vi "TestLoop ReadDataAndSwitchBuffers.vi"() -> ()   [LabVIEW 2013]
uses:
  My circular buffer info.ctl
panel:
  out "buffer size (in bytes)":i64
  out "Buffer offset (in bytes)":i64
  out "element read buffer Q":refnum<file>
  out "elements of read buffer Q":refnum<file>[](array[refnum])
  out "# elements in read buffer Q":i32
  out "element command Q":enum16{"toggle buffers", "data event", "stop"}(ring)
  out "elements command Q":enum16{"toggle buffers", "data event", "stop"}[](array[ring])
  out "# elements in command Q":i32
  in  "stop":bool
  in  "buffer2 path":path
  in  "buffer1 path":path
  in  "archive directory":path
  in  "num blocks  prior":i32
  in  "num blocks after":i32
  in  "bytes/sample":i32
  in  "samples/block/channel":i32
  in  "number of channels":i32
  out "write pointer (block position)":i32
  out "Waveform Graph":i16[][](graph)
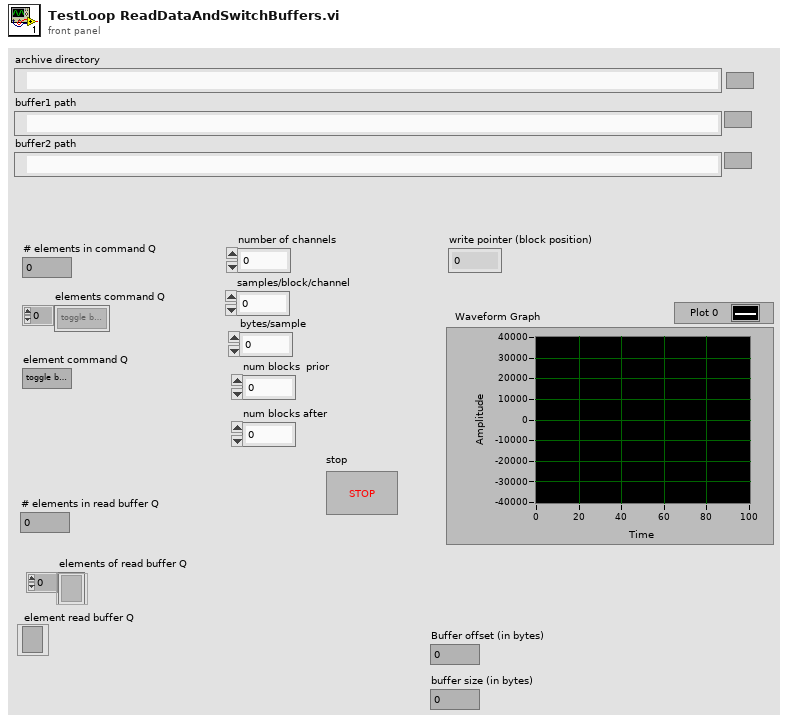
[diagram p1: front panel]
types:
  T1 = typedef "My circular buffer info.ctl" = cluster{"buff ref1":refnum<file>, "buff ref2":refnum<file>, "buffer1 path":path, "buffer2 path":path, "archive directory":path, "xml header":string, "num blocks  prior":i32, "num blocks after":i32, "blocks/event":i32, "samples/block":i32, "bytes/sample":i32, "number of channels":i32, "samples/block/channel":i32, "read buffer ref queue":refnum<queue>, "Event delay queue":refnum<queue>, "command queue":refnum<queue>}
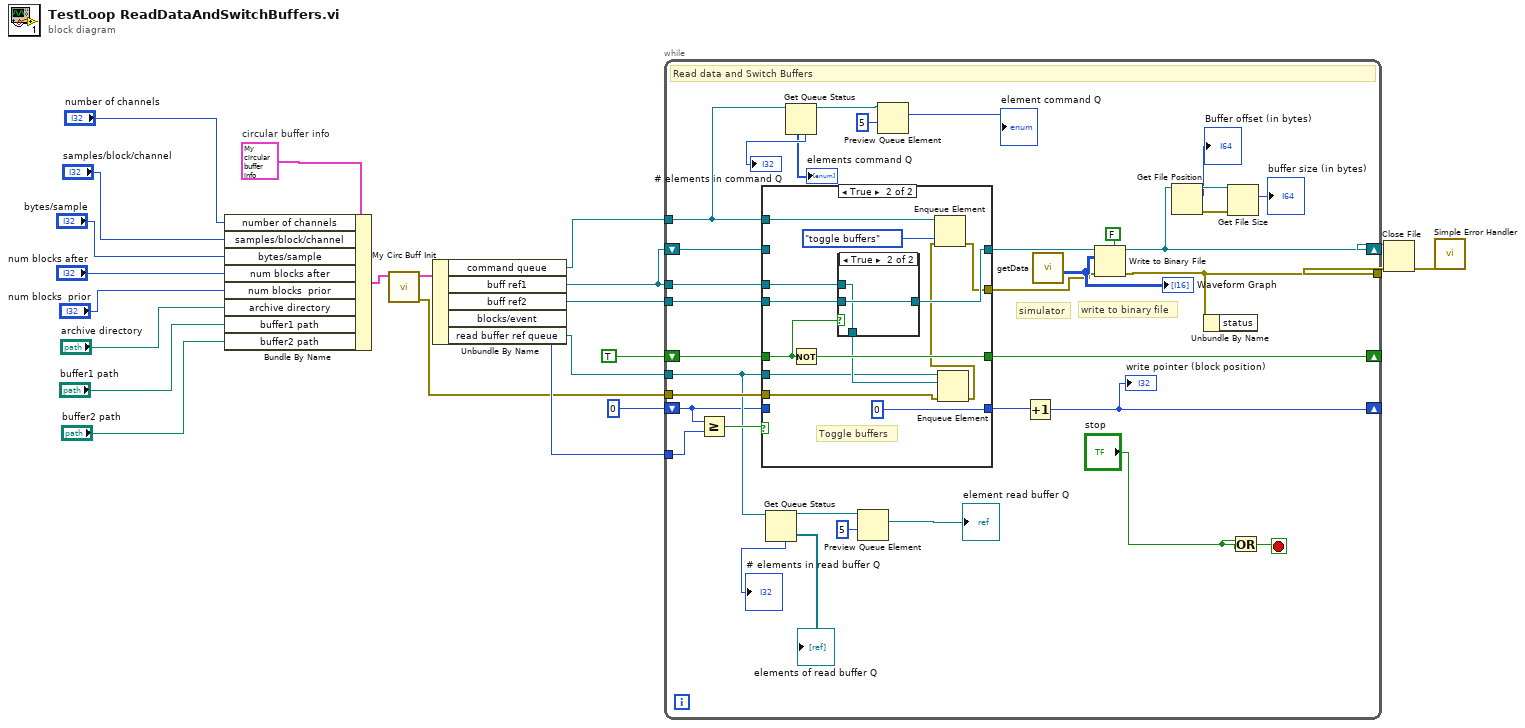
[diagram p0: block diagram]
diagram:
  w17 = T1 {"buff ref1"=refnum, "buff ref2"=refnum, "buffer1 path"=path "", "buffer2 path"=path "", "archive directory"=path "", "xml header"="", "num blocks  prior"=0, "num blocks after"=0, "blocks/event"=0, "samples/block"=0, "bytes/sample"=0, "number of channels"=0, "samples/block/channel"=0, "read buffer ref queue"=refnum, "Event delay queue"=refnum, "command queue"=refnum}  # circular buffer info
  n1 = Bundle By Name(cluster=w17, "number of channels"="number of channels", "samples/block/channel"="samples/block/channel", "bytes/sample"="bytes/sample", "num blocks after"="num blocks after", "num blocks  prior"="num blocks  prior", "archive directory"="archive directory", "buffer1 path"="buffer1 path", "buffer2 path"="buffer2 path") -> (w13:T1)
  n2 = call "My Circ Buff Init.vi"("circular buffer info"=w13) -> ("error out"=w4:errorcluster, "circular buffer info out"=w5:T1)  [unwired: 9 in]
  n3 = Unbundle By Name(w5) -> ("command queue"=w6:refnum<queue>, "buff ref1"=w8:refnum<file>, "buff ref2"=w10:refnum<file>, "blocks/event"=w12:i32, "read buffer ref queue"=w7:refnum<queue>)
  n4 = while {
    tunnel: w12 -> [w56]
    shift-right: [w53] -> _
    shift-left: 0 -> [w29]
    shift-right: [w26] -> w3
    shift-left: w8 -> [w51]
    tunnel: w10 -> [w50]
    shift-right: [w48] -> _
    shift-left: TRUE -> [w49]
    tunnel: w8 -> [w47]
    tunnel: w7 -> [w36]
    tunnel: w6 -> [w41]
    tunnel: w4 -> [w45]
    tunnel: [w42] -> w2
    stop <- w43 stop-if-true
    # "simulator"
    # "write to binary file"
    # "Read data and Switch Buffers"
    n5 = Greater Or Equal?(x=w29, y=w56) -> (x >= y?=w55:bool)
    n6 = case shown="True" w55 {
      tunnel: w29 -> [w61 _]
      tunnel: [w61 0] -> w54
      tunnel: [w60 w71] -> w52
      tunnel: w51 -> [w60 _]
      tunnel: w50 -> [_ w72]
      tunnel: w49 -> [w59 w73]
      tunnel: [w59 w74] -> w48
      tunnel: w47 -> [_ w70]
      tunnel: w36 -> [_ w68]
      tunnel: w41 -> [_ w67]
      tunnel: w45 -> [w58 w65]
      tunnel: [w58 w63] -> w44
      frame False {
      }
      frame True {
        # "Toggle buffers"
        n7 = Not(x=w73) -> (.not. x?=w74:bool)
        n8 = case shown="True" w73 {
          tunnel: w72 -> [w75 w78]
          tunnel: [w76 w78] -> w71
          tunnel: w70 -> [w76 w77]
          tunnel: [w75 w77] -> w69
          frame False {
          }
          frame True {
          }
        }
        n9 = Enqueue Element(queue=w68, element=w69, error in (no error)=w65) -> (error out=w64:errorcluster)  [unwired: 1 in, 2 out]
        n10 = Enqueue Element(queue=w67, element=enum16{"toggle buffers", "data event", "stop"}."toggle buffers", error in (no error)=w64) -> (error out=w63:errorcluster)  [unwired: 1 in, 2 out]
      }
    }
    n11 = Get Queue Status(queue=w36) -> (queue out=w35:refnum<queue>, # elements in queue=→"# elements in read buffer Q":i32, elements=→"elements of read buffer Q":refnum<file>[])  [unwired: 2 in, 5 out]
    n12 = Get Queue Status(queue=w41) -> (queue out=w40:refnum<queue>, # elements in queue=→"# elements in command Q":i32, elements=→"elements command Q":enum16{"toggle buffers", "data event", "stop"}[])  [unwired: 2 in, 5 out]
    n13 = Preview Queue Element(queue=w35, timeout in ms (-1)=5) -> (element=→"element read buffer Q":refnum<file>)  [unwired: 1 in, 3 out]
    n14 = Preview Queue Element(queue=w40, timeout in ms (-1)=5) -> (element=→"element command Q":enum16{"toggle buffers", "data event", "stop"})  [unwired: 1 in, 3 out]
    n15 = Increment(x=w54) -> (x+1=w53:i32)
    "write pointer (block position)" <- w53
    n16 = call "getData.vi"() -> ("binary data"=w46:i16[][])  [unwired: 7 in]
    "Waveform Graph" <- w46
    n17 = Write to Binary File(file (use dialog)=w52, data=w46, error in=w44, 5:FALSE ("prepend array or string size? (T)")) -> (refnum out=w26:refnum<file>, error out=w42:errorcluster)  [unwired: 2 in, 1 out]
    n18 = Get File Position(7:w26) -> (0:w27:errorcluster, 2:→"Buffer offset (in bytes)":i64, 3:w25:refnum<file>)  [unwired: 1 in]
    n19 = Unbundle By Name(w42) -> ()  [unwired: 1 out]
    n20 = Get File Size(file=w25, error in=w27) -> (size (in bytes)=→"buffer size (in bytes)":i64)  [unwired: 2 out]
    n21 = Or(x="stop", y="stop") -> (x .or. y?=w43:bool)
  }
  n22 = Close File(refnum=w3, error in=w2) -> (error out=w1:errorcluster)  [unwired: 1 out]
  n23 = call <vilib>:"Simple Error Handler.vi"("error in (no error)"=w1) -> ()  [unwired: 4 in, 5 out]
